vi "PH_USB600x_AnalogReader.ProcPeriodic.vi"(0 "i ref in":refnum<vi>, 3 "ms timeout (10000)":i32=10000, 5 "error in (no error)":errorcluster) -> (14 "i ref out":refnum<vi>, 17 "timed out":bool, 19 "error out":errorcluster)   [LabVIEW 2014, in "PH_USB600x_AnalogReader.lvlib"]
doc: "This method serves to periodically do things like reading values from the HW. Methods that should be executed periodically should be called from THIS methode. Add code here."
uses:
  PH_USB600x_AnalogReader.lvlib
  CSCore/BaseProcess/BaseProcess.lvlib
  CSCore/CSSystem/CSSystemLib/CSSystemLib.lvlib
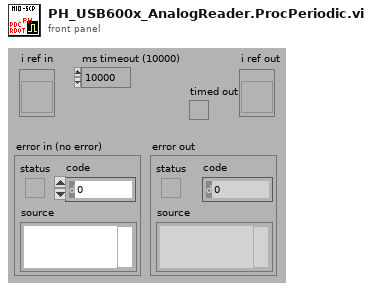
[diagram p1: front panel]
types:
  T1 = typedef "PH_USB600x_AnalogReader.lvlib/PH_USB600x_AnalogReader.i attribute.ctl" = cluster{"GUI Refs":cluster{"Delete":refnum<vi>, "Status":refnum<vi>, "Timeout":refnum<vi>, "Acquire Waveform":refnum<vi>, "Timing":refnum<vi>, "Graph":refnum<vi>, "Prdc Interval":refnum<vi>, "Formula":refnum<vi>}, "Device Settings":cluster{"AIChannel":refnum<k21>, "channelName":string, "Status":T2}, "Timing":T3, "Prdc Interval":dbl, "Lin Scaling":T4, "Data":cluster{"t0":timestamp, dbl}[]}
  T2 = typedef "PH_StatusHandler.lvlib/PH_StatusHandler.Status.ctl" = i16
  T3 = typedef "PH_USB600x_AnalogReader.lvlib/PH_USB600x_AnalogReader.Timing.ctl" = cluster{"Samples per Channel":i32, "Rate":dbl}
  T4 = typedef "PH_USB600x_AnalogReader.lvlib/PH_USB600x_AnalogReader.Lin Scaling.ctl" = cluster{"Slope [Unit/V]":dbl, "Offset [Unit]":dbl, "Y-Unit":string, "Y-Label":string}
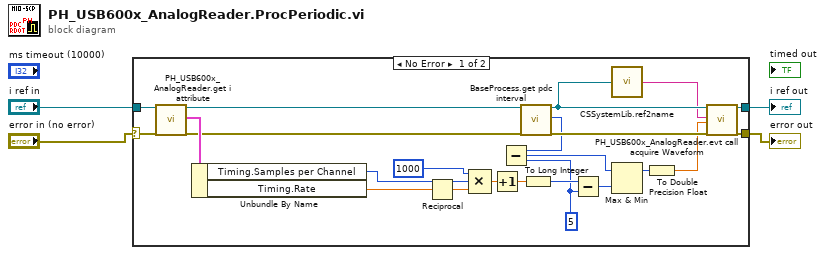
[diagram p0: block diagram]
diagram:
  n1 = case shown="No Error" "error in (no error)" {
    selector: "error in (no error)" -> [w27 w28]
    tunnel: [w17 w28] -> w1
    tunnel: "i ref in" -> [w26 w29]
    tunnel: [w16 w29] -> w2
    frame No Error {
      w11 = 5 ("y")
      n2 = call "PH_USB600x_AnalogReader.get i attribute.vi"("i ref in"=w26, "error in (no error)"=w27) -> ("i ref out"=w24:refnum<vi>, "i attribute"=w25:T1, "error out"=w23:errorcluster)  [unwired: 15 in]
      n3 = Unbundle By Name(w25) -> ("Timing.Samples per Channel"=w7:i32, "Timing.Rate"=w20:dbl)
      n4 = Reciprocal(x=w20) -> (1/x=w21:dbl)
      n5 = Compound Arithmetic op=MULTIPLY(1000 ("value"), w7, w21) -> (w22:dbl)
      n6 = Increment(x=w22) -> (x+1=w19:dbl)
      n7 = call "BaseProcess.get pdc interval.vi"("i ref in"=w24, "error in (no error)"=w23) -> ("i ref out"=w15:refnum<vi>, "PeriodicInterval"=w13:i32, "error out"=w18:errorcluster)  [unwired: 15 in]
      n8 = Subtract(x=w13, y=w11) -> (x-y=w9:i32)
      n9 = To Long Integer(number=w19) -> (32bit integer=w12:i32)
      n10 = Subtract(x=w12, y=w11) -> (x-y=w10:i32)
      n11 = call "CSSystemLib.ref2name.vi"("obj refnum"=w15) -> ("name"=w14:string)
      n12 = Max & Min(x=w9, y=w10) -> (max(x,y)=w6:i32)  [unwired: 1 out]
      n13 = To Double Precision Float(number=w6) -> (double precision float=w5:dbl)
      n14 = call "PH_USB600x_AnalogReader.evt call acquire Waveform.vi"("i ref in"=w15, "Instance"=w14, "Timeout"=w5, "error in"=w18) -> ("i ref out"=w16:refnum<vi>, "error out"=w17:errorcluster)  [unwired: 14 in]
    }
    frame Error {
    }
  }
  "error out" <- w1
  "i ref out" <- w2
